vi "Set Tuner Gain Mode.vi"(8 "error in (no error)":errorcluster, 10 "AutoGain":bool, 11 "DeviceRefnum":u64) -> (0 "error out":errorcluster, 2 "function return":i32, 3 "DeviceRefnum Out":u64)   [LabVIEW 2014]
doc: "Set the gain mode (automatic/manual) for the device. Manual gain mode must be enabled for the gain setter function to work."
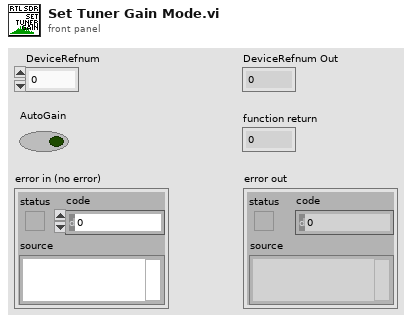
[diagram p1: front panel]
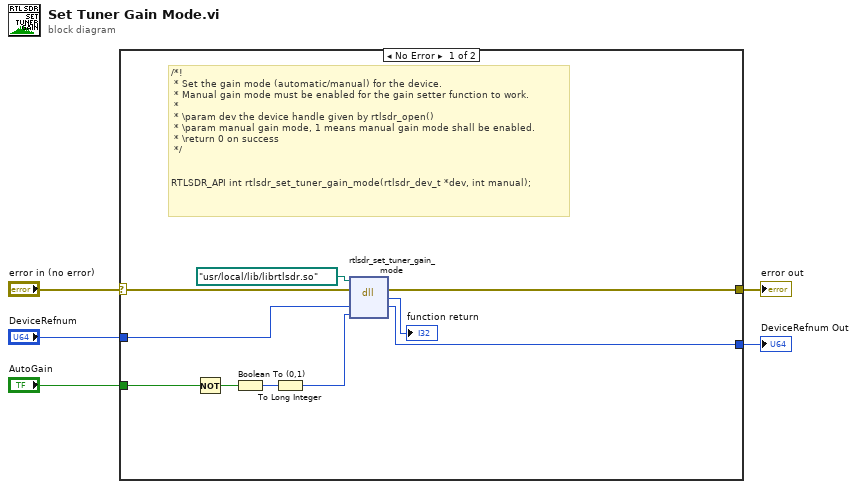
[diagram p0: block diagram]
diagram:
  n1 = case shown="No Error" "error in (no error)" {
    selector: "error in (no error)" -> [w6 w17]
    tunnel: [w14 w17] -> w5
    tunnel: "DeviceRefnum" -> [w13 w16]
    tunnel: [w12 w16] -> w3
    tunnel: "AutoGain" -> [w11 _]
    frame No Error {
      # "/*!\n * Set the gain mode (automatic/manual) for the device.\n * Manual gain mode must be enabled for the gain setter function to work.\n *\n * \\param dev the device handle given by rtlsdr_open()\n * \\param manual gain mode, 1 means manual gain mode shall be enabled.\n * \\return 0 on success\n */\n\n\nRTLSDR_API int rtlsdr_set_tuner_gain_mode(rtlsdr_dev_t *dev, int manual);"
      n2 = Not(x=w11) -> (.not. x?=w10:bool)
      n3 = Boolean To (0,1)(Boolean=w10) -> (0, 1=w9:i16)
      n4 = To Long Integer(number=w9) -> (32bit integer=w8:i32)
      n5 = dll-call lib="C:/Program Files (x86)/National Instruments/LabVIEW 2016/user.lib/rtlsdr/rtlsdr.*" fn="rtlsdr_set_tuner_gain_mode"(path in=path "/usr/local/lib/librtlsdr.so", error in=w6, "DeviceRefnum"=w13, "GainMode"=w8) -> (error out=w14:errorcluster, "return type"=→"function return":i32, "DeviceRefnum"=w12:u64)  [unwired: 2 in, 1 out]
    }
    frame Error {
    }
  }
  "error out" <- w5
  "DeviceRefnum Out" <- w3
